vi "switch - C.vi"(9 "switch":bool=TRUE) -> (1 "result":bool=TRUE)   [LabVIEW 2015]
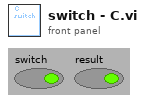
[diagram p1: front panel]
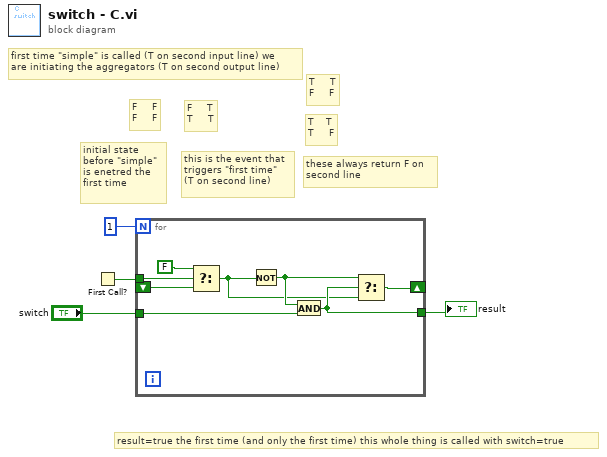
[diagram p0: block diagram]
diagram:
  # "result=true the first time (and only the first time) this whole thing is called with switch=true"
  # "these always return F on \nsecond line"
  # "initial state\nbefore \"simple\"\nis enetred the \nfirst time"
  # "this is the event that \ntriggers \"first time\" \n(T on second line)"
  # "F     F\nF     F"
  # "T     T\nF     F"
  # "F     T\nT     T"
  # "T    T\nT     F"
  # "first time \"simple\" is called (T on second input line) we \nare initiating the aggregators (T on second output line)"
  n1 = First Call?() -> (First Call?: T/F=w2:bool)
  n2 = for {
    N: 1 -> [_]
    tunnel: "switch" -> [w11]
    tunnel: [w9] -> w3
    shift-right: [w10] -> _
    shift-left: _ -> [w6]
    tunnel: w2 -> [w8]
    n3 = Select(t=FALSE, s=w8, f=w6) -> (s? t:f=w5:bool)
    n4 = Not(x=w5) -> (.not. x?=w12:bool)
    n5 = And(x=w12, y=w11) -> (x .and. y?=w9:bool)
    n6 = Select(t=w12, s=w9, f=w5) -> (s? t:f=w10:bool)
  }
  "result" <- w3
